vi "Get Acyclic Frame from Trigger.vi"(8 "error in":errorcluster, 11 "acyclic frame trigger":T2 format="%.0x") -> (0 "error out":errorcluster, 2 "acyclic frame out":T1, 3 "acyclic frame trigger out":T2 format="%.0x", 4 "found?":bool)   [LabVIEW 2020, in "AIM MIL-STD-1553 Scripting.lvlib"]
doc: "Returns the <b>acyclic frame out</b> and its messages for the specified <b>acyclic frame trigger</b>."
uses:
  AIM MIL-STD-1553 Scripting.lvlib
  <vilib>/NI VeriStand/Custom Device API/Custom Device Item Ref.ctl
  Constants.vi
  <vilib>/NI VeriStand/Custom Device API/Get Item Property (String).vi
  <vilib>/NI VeriStand/Custom Device API/Custom Device API.lvlib
  Shared/Acyclic Frame Definition.ctl
  <vilib>/NI VeriStand/Custom Device API/Get Item Property (String Array).vi
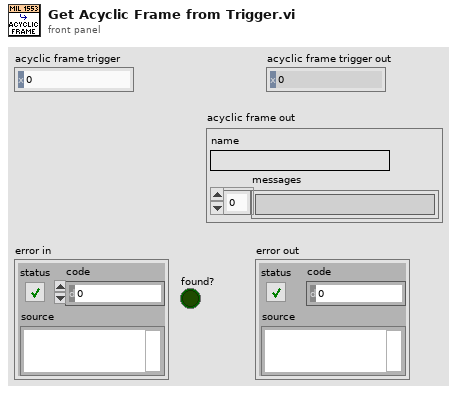
[diagram p1: front panel]
types:
  T1 = typedef "Acyclic Frame Definition.ctl" = cluster{"name":string, "messages":string[]}
  T2 = typedef "Custom Device API.lvlib/Custom Device Item Ref.ctl" = u64
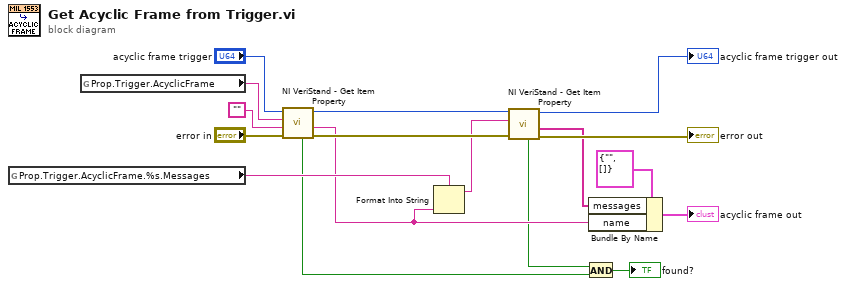
[diagram p0: block diagram]
diagram:
  n1 = global read "Constants.vi" "Prop.Trigger.AcyclicFrame.%s.Messages"() -> (w8:string)
  n2 = global read "Constants.vi" "Prop.Trigger.AcyclicFrame"() -> (w17:string)
  n3 = call-poly <vilib>:"NI VeriStand - Get Item Property.vi"("error in (no error)"="error in", "Default Value"="", "Property Name"=w17, "Item Ref in"="acyclic frame trigger") -> ("error out"=w12:errorcluster, "Value"=w7:string, "Item Ref out"=w10:T2, "Found?"=w2:bool)  [unwired: 4 in]
  n4 = Format Into String(format string=w8, w7) -> (resulting string=w6:string)  [unwired: 2 in, 1 out]
  n5 = call-poly <vilib>:"NI VeriStand - Get Item Property.vi"("error in (no error)"=w12, "Property Name"=w6, "Item Ref in"=w10) -> ("error out"=→"error out":errorcluster, "Value"=w5:string[], "Item Ref out"=→"acyclic frame trigger out":T2, "Found?"=w3:bool)  [unwired: 5 in]
  n6 = And(x=w3, y=w2) -> (x .and. y?=→"found?":bool)
  n7 = Bundle By Name(cluster=T1 {"name"="", "messages"=[]} ("acyclic frame out"), "messages"=w5, "name"=w7) -> (→"acyclic frame out":T1)
